vi "score sorter.vi"(11 "Array in":dbl[](array[numeric])) -> (1 "Array out":dbl[](array[numeric]), 2 "Numeric 2":dbl, 3 "Numeric":dbl)   [LabVIEW 2014]
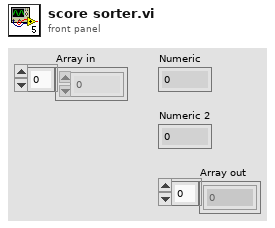
[diagram p1: front panel]
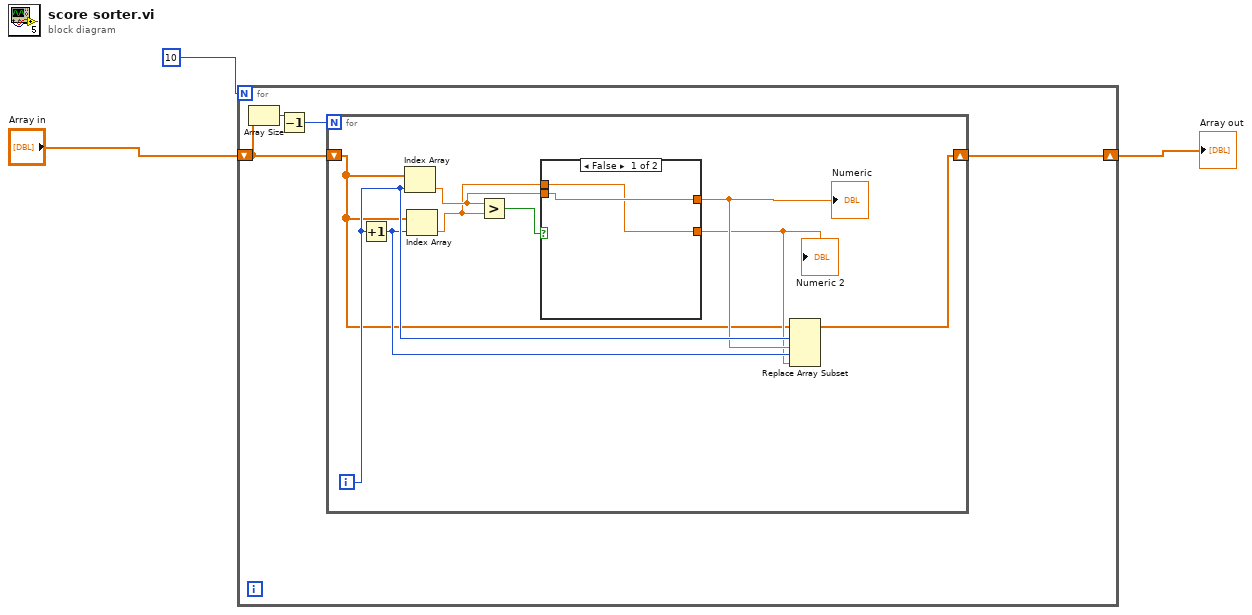
[diagram p0: block diagram]
diagram:
  n1 = for {
    N: 10 -> [_]
    shift-right: [w5] -> w3
    shift-left: "Array in" -> [w4]
    n2 = Array Size(array=w4) -> (size(s)=w7:i32)
    n3 = Decrement(x=w7) -> (x-1=w6:i32)
    n4 = for {
      N: w6 -> [_]
      shift-right: [w8] -> w5
      shift-left: w4 -> [w9]
      i -> [w13]
      n5 = Increment(x=w13) -> (x+1=w11:i32)
      n6 = Index Array(array=w9, index=w13) -> (element=w15:dbl)
      n7 = Index Array(array=w9, index=w11) -> (element=w14:dbl)
      n8 = Greater?(x=w15, y=w14) -> (0:w16:bool)
      n9 = case shown="False" w16 {
        tunnel: [w17 w20] -> w10
        tunnel: w15 -> [w18 w20]
        tunnel: [w18 w19] -> w12
        tunnel: w14 -> [w17 w19]
        frame False {
        }
        frame True {
        }
      }
      "Numeric" <- w12
      "Numeric 2" <- w10
      n10 = Replace Array Subset(array=w9, new element #1=w12, index #1=w13, new element #2=w10, index #2=w11) -> (w8:dbl[])
    }
  }
  "Array out" <- w3
